vi "Read_obs_files.vi"(0 "Path":path) -> (1 "path used":path, 2 "Output Table":string[][](array[string]))   [LabVIEW 2011]
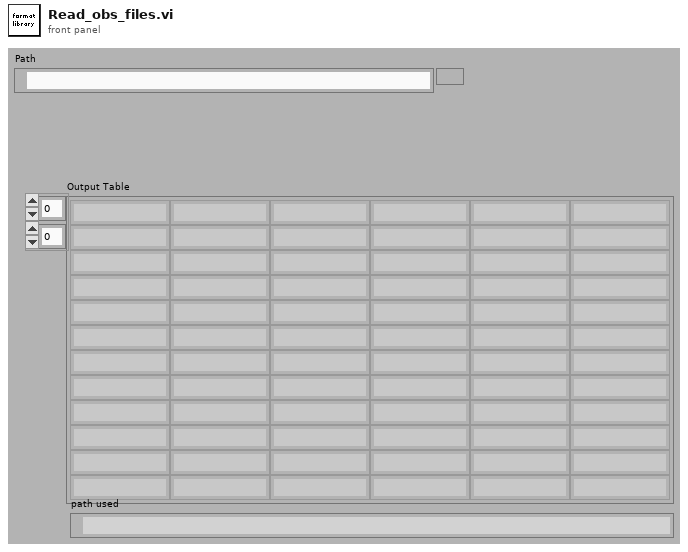
[diagram p1: front panel]
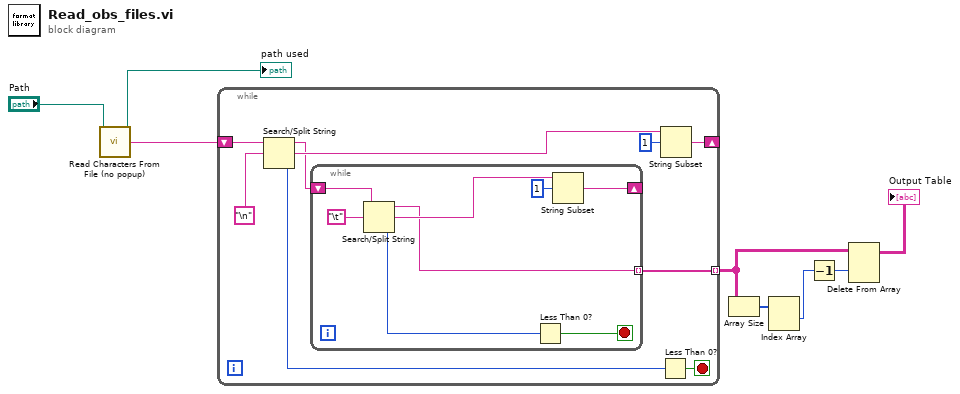
[diagram p0: block diagram]
diagram:
  n1 = call "Read Characters From File (no popup).vi"("file path (dialog if empty)"="Path") -> ("new file path (NotAPath if cancelled)"=→"path used":path, "character string"=w7:string)  [unwired: 5 in, 2 out]
  n2 = while {
    shift-right: [w16] -> _
    shift-left: w7 -> [w17]
    tunnel: [w10] -> w5 mode=indexing
    stop <- w11 stop-if-true
    n3 = Search/Split String(string=w17, search string/char (-)="\n") -> (substring before match=w13:string, match + rest of string=w14:string, offset of match=w12:i32)  [unwired: 1 in]
    n4 = while {
      shift-right: [w21] -> _
      shift-left: w13 -> [w24]
      tunnel: [w20] -> w10 mode=indexing
      stop <- w19 stop-if-true
      n5 = Search/Split String(string=w24, search string/char (-)="\t") -> (substring before match=w20:string, match + rest of string=w22:string, offset of match=w18:i32)  [unwired: 1 in]
      n6 = Less Than 0?(x=w18) -> (x < 0?=w19:bool)
      n7 = String Subset(string=w22, offset (0)=1) -> (substring=w21:string)  [unwired: 1 in]
    }
    n8 = Less Than 0?(x=w12) -> (x < 0?=w11:bool)
    n9 = String Subset(string=w14, offset (0)=1) -> (substring=w16:string)  [unwired: 1 in]
  }
  n10 = Array Size(array=w5) -> (size(s)=w6:i32[])
  n11 = Index Array(array=w6) -> (element #1=w4:i32)  [unwired: 2 in, 1 out]
  n12 = Decrement(x=w4) -> (x-1=w2:i32)
  n13 = Delete From Array(array=w5, index (row)=w2) -> (array with subset deleted=→"Output Table":string[][])  [unwired: 2 in, 1 out]
